vi "Package GroupData Msg.vi"(8 "error in (no error)":errorcluster, 11 "Group in":refnum<class "Group.lvclass">) -> (0 "error out":errorcluster, 2 "GroupData":refnum<class "Msg.lvclass">, 3 "Group out":refnum<class "Group.lvclass">)   [LabVIEW 2020, in "Vecto.lvlib" / "Group.lvclass"]
uses:
  Group.lvclass
  proto/GroupData/Class/Msg.lvclass
  Group.lvclass/Group.ctl
  proto/GroupData/Data.ctl
  proto/GroupData/Class/Msg.lvclass/Msg.ctl
  proto/GroupData/GroupData.lvlib
  Vecto.lvlib
  Group Config/Group Config.lvclass
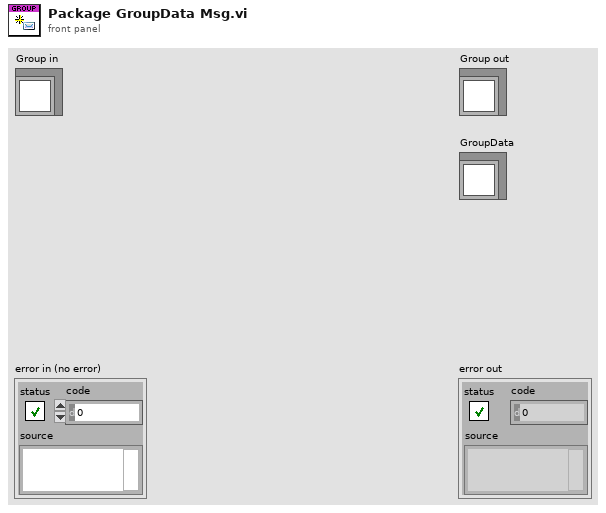
[diagram p1: front panel]
types:
  T1 = typedef "GroupData.lvlib/Data.ctl" = cluster{"group_name":string, "data_timestamp":i64, "scaled_data":dbl[], "raw_data":dbl[]}
  T2 = typedef "Vecto.lvlib/Group.lvclass/Ref.ctl" = cluster{"Channel Index Map":map{string, i32}, "Channel Info":T3[], "Channel Value":T4[]}
  T3 = typedef "Vecto.lvlib/Channel Info.ctl" = cluster{"Name":string, "Group":string, "Owning Node":u32, "Owning Task":u32, "Resource":string}
  T4 = typedef "Vecto.lvlib/Channel Value.ctl" = cluster{"Scaled":dbl, "Timestamp":dbl, "Raw":dbl}
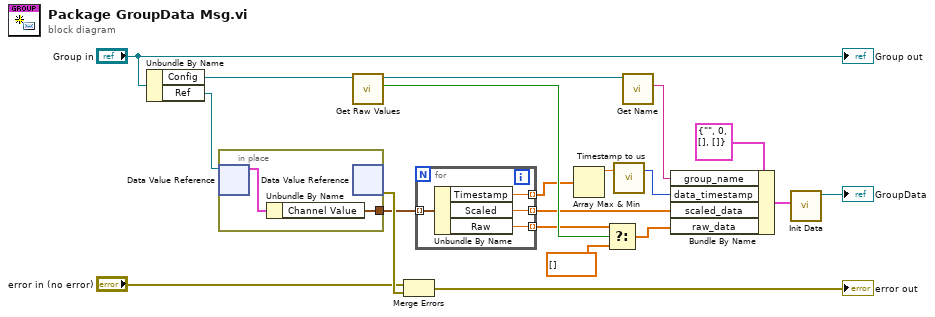
[diagram p0: block diagram]
diagram:
  n1 = Unbundle By Name("Group in") -> ("Config"=w10:refnum<class "Group Config.lvclass">, "Ref"=w17:refnum<data-value>)
  n2 = in-place {
    in-place-border: [w21] -> w4
    n3 = in-place-dvr #1(w17) -> (w22:T2)  [unwired: 1 out]
    n4 = Unbundle By Name(w22) -> ("Channel Value"=w21:T4[])
    n5 = in-place-dvr #1() -> (w20:errorcluster)  [unwired: 1 in, 1 out]
  }
  n6 = call "Get Raw Values.vi"("Group Config in"=w10) -> ("Raw Values"=w9:bool, "Group Config out"=w8:refnum<class "Group Config.lvclass">)  [unwired: 8 in, 1 out]
  n7 = Merge Errors("error in (no error)", w20) -> (→"error out":errorcluster)
  n8 = for {
    tunnel: w4 -> [w23] mode=indexing
    tunnel: [w26] -> w3 mode=indexing
    tunnel: [w25] -> w2 mode=indexing
    tunnel: [w24] -> w1 mode=indexing
    n9 = Unbundle By Name(w23) -> ("Timestamp"=w26:dbl, "Scaled"=w25:dbl, "Raw"=w24:dbl)
  }
  n10 = Array Max & Min(array=w3) -> (max value=w15:dbl)  [unwired: 3 out]
  n11 = Select(t=w1, s=w9, f=dbl[] []) -> (s? t:f=w11:dbl[])
  n12 = call "Timestamp to us.vi"("Timestamp"=w15) -> ("Timestamp us"=w14:i64)  [unwired: 6 in]
  n13 = call "Get Name.vi"("Group Config in"=w8) -> ("Name"=w7:string)  [unwired: 8 in, 2 out]
  n14 = Bundle By Name(cluster=T1 {"group_name"="", "data_timestamp"=0, "scaled_data"=[], "raw_data"=[]} ("GroupData"), "group_name"=w7, "data_timestamp"=w14, "scaled_data"=w2, "raw_data"=w11) -> (w6:T1)
  n15 = call "Init Data.vi"("Data"=w6) -> ("Msg out"=→"GroupData":refnum<class "Msg.lvclass">)  [unwired: 10 in]
  "Group out" <- "Group in"
